vi "BRig_dataTrial_T_Cue2_Audio.vi"() -> (2 "output_T_Cue2_Audio":i32)   [LabVIEW 2014]
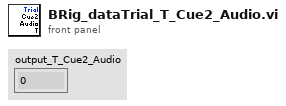
[diagram p1: front panel]
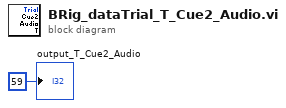
[diagram p0: block diagram]
diagram:
  "output_T_Cue2_Audio" <- 59 ("output_iBlock")
